vi "PDC Start Data Stream.vi"(8 "error in (no error)":errorcluster, 11 "Phasor Data Concentrator in":refnum<class "Phasor Data Concentrator.lvclass">) -> (0 "error out":errorcluster, 3 "Phasor Data Concentrator out":refnum<class "Phasor Data Concentrator.lvclass">)   [LabVIEW 2013, in "PMU Recorder Light.lvlib" / "Phasor Data Concentrator.lvclass"]
uses:
  Phasor Data Concentrator.lvclass
  Phasor Data Concentrator.lvclass/Phasor Data Concentrator.ctl
  Statnett C37.118 DLL/Statnett C37.118 DLL.lvclass
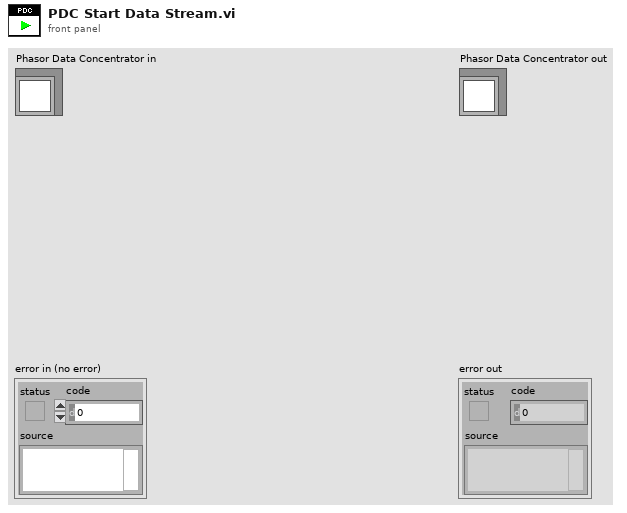
[diagram p1: front panel]
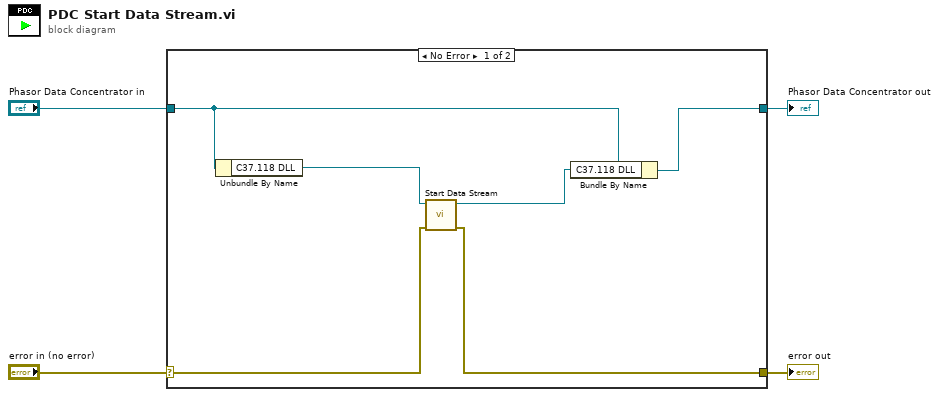
[diagram p0: block diagram]
diagram:
  n1 = case shown="No Error" "error in (no error)" {
    selector: "error in (no error)" -> [w6 w12]
    tunnel: [w5 w12] -> w3
    tunnel: [w9 w11] -> w1
    tunnel: "Phasor Data Concentrator in" -> [w10 w11]
    frame No Error {
      n2 = Unbundle By Name(w10) -> ("C37.118 DLL"=w7:refnum<class "Statnett C37.118 DLL.lvclass">)
      n3 = call "Start Data Stream.vi"("error in (no error)"=w6, "Statnett C37.118 DLL in"=w7) -> ("error out"=w5:errorcluster, "Statnett C37.118 DLL out"=w8:refnum<class "Statnett C37.118 DLL.lvclass">)  [unwired: 8 in]
      n4 = Bundle By Name(cluster=w10, "C37.118 DLL"=w8) -> (w9:refnum<class "Phasor Data Concentrator.lvclass">)
    }
    frame Error {
    }
  }
  "error out" <- w3
  "Phasor Data Concentrator out" <- w1
